vi "Find RT Projects.vi"() -> (1 "Paths":path[](array[path]), 2 "Targets":refnum<vi>[](array[refnum]), 3 "Project Names":string[](array[string]))   [LabVIEW 2023]
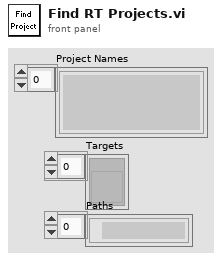
[diagram p1: front panel]
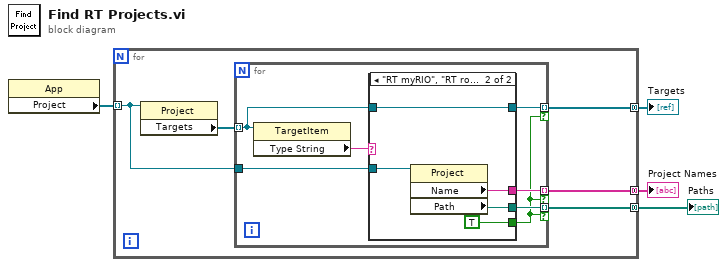
[diagram p0: block diagram]
diagram:
  n1 = property class="App"() -> ("Project"=w4:refnum<vi>[])  [unwired: 2 in, 2 out]
  n2 = for {
    tunnel: w4 -> [w8] mode=indexing
    tunnel: [w7] -> w3 mode=concatenating
    tunnel: [w6] -> w2 mode=concatenating
    tunnel: [w5] -> w1 mode=concatenating
    n3 = property class="Project"(reference=w8) -> ("Targets"=w9:refnum<vi>[])  [unwired: 1 in, 2 out]
    n4 = for {
      tunnel: w9 -> [w13] mode=indexing
      tunnel: w8 -> [w15]
      tunnel: [w14] -> w7 mode=indexing if=w10
      tunnel: [w12] -> w6 mode=indexing if=w10
      tunnel: [w11] -> w5 mode=indexing if=w10
      n5 = property class="TargetItem"(reference=w13) -> ("Type String"=w16:string)  [unwired: 1 in, 2 out]
      n6 = case shown="\"RT myRIO\", \"RT roboRIO\"" w16 {
        tunnel: w15 -> [_ w21]
        tunnel: [_ w20] -> w14
        tunnel: [_ TRUE] -> w10
        tunnel: w13 -> [_ w18]
        tunnel: [_ w18] -> w12
        tunnel: [_ w17] -> w11
        frame Default {
        }
        frame "RT myRIO", "RT roboRIO" {
          n7 = property class="Project"(reference=w21) -> ("Name"=w20:string, "Path"=w17:path)  [unwired: 1 in, 2 out]
        }
      }
    }
  }
  "Project Names" <- w3
  "Targets" <- w2
  "Paths" <- w1
